vi "stimulus_intensity_to_red_blue_color.vi"(1 "StimulusIntensityForFrame":sgl[](array[numeric])) -> (0 "StimulusColorForFrame":sgl[](array[numeric]))   [LabVIEW 2019]
uses:
  ParametersGlobal.vi
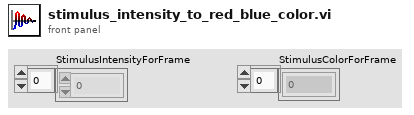
[diagram p1: front panel]
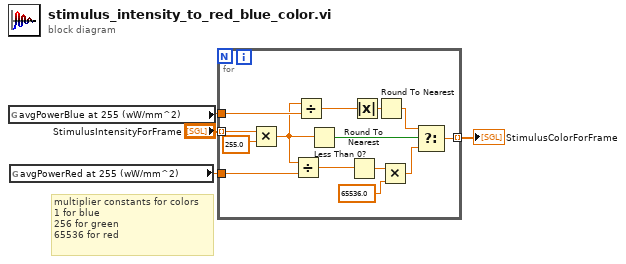
[diagram p0: block diagram]
diagram:
  # "multiplier constants for colors\n1 for blue\n256 for green\n65536 for red"
  n1 = global read "ParametersGlobal.vi" "avgPowerBlue at 255 (wW/mm^2)"() -> (w2:sgl)
  n2 = global read "ParametersGlobal.vi" "avgPowerRed at 255 (wW/mm^2)"() -> (w1:sgl)
  n3 = for {
    tunnel: "StimulusIntensityForFrame" -> [w7] mode=indexing
    tunnel: [w14] -> w3 mode=indexing
    tunnel: w2 -> [w11]
    tunnel: w1 -> [w10]
    n4 = Multiply(x=w7, y=sgl 255.0) -> (x*y=w6:sgl)
    n5 = Divide(x=w6, y=w10) -> (x/y=w9:sgl)
    n6 = Divide(x=w6, y=w11) -> (x/y=w8:sgl)
    n7 = Less Than 0?(x=w6) -> (x < 0?=w18:bool)
    n8 = Round To Nearest(number=w9) -> (nearest integer value=w16:sgl)
    n9 = Absolute Value(x=w8) -> (abs(x)=w13:sgl)
    n10 = Round To Nearest(number=w13) -> (nearest integer value=w12:sgl)
    n11 = Multiply(x=w16, y=sgl 65536.0) -> (x*y=w15:sgl)
    n12 = Select(t=w12, s=w18, f=w15) -> (s? t:f=w14:sgl)
  }
  "StimulusColorForFrame" <- w3
